vi "UIManager.GetBroadcasts.vi"(11 "NewTemplate in":refnum<class "UIManager.lvclass">) -> (2 "TemplateModule":cluster{"Broadcasts":T1, "Broadcasts":T2}, 3 "NewTemplate out":refnum<class "UIManager.lvclass">)   [LabVIEW 2024, in "UIManager.lvclass"]
uses:
  UIManager.lvclass
  UIManager.lvclass/UIManager.ctl
  RQMHCore/ModuleCore/RQMHModule.lvclass
  RQMHCore/Shared/Died.ctl
  RQMHCore/Shared/RQMHShared.lvlib
  RQMHCore/ModuleCore/StandardBroadcasts.ctl
  Stopped.ctl
  Broadcast Events--cluster.ctl
  RQMHCore/ModuleCore/Started.ctl
  Request Stop.ctl
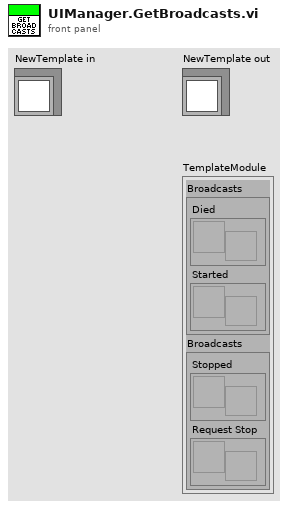
[diagram p1: front panel]
types:
  T1 = typedef "RQMHModule.lvclass/StandardBroadcasts.ctl" = cluster{"Died":refnum<user-event>, "Started":refnum<user-event>}
  T2 = typedef "UIManager.lvclass/Broadcast Events--cluster.ctl" = cluster{"Stopped":refnum<user-event>, "Request Stop":refnum<user-event>}
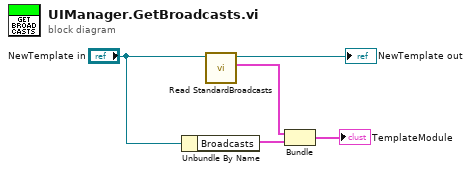
[diagram p0: block diagram]
diagram:
  n1 = Unbundle By Name("NewTemplate in") -> ("Broadcasts"=w5:T2)
  n2 = call "Read StandardBroadcasts.vi"("JQMHCore in"="NewTemplate in") -> ("Broadcasts"=w4:T1, "JQMHCore out"=→"NewTemplate out":refnum<class "UIManager.lvclass">)  [unwired: 8 in, 1 out]
  n3 = Bundle("Broadcasts"=w4, "Broadcasts"=w5) -> (→"TemplateModule":cluster{"Broadcasts":T1, "Broadcasts":T2})  [unwired: 1 in]
